vi "FetchSettings.vi"(3 "error in (no error)":errorcluster, 5 "resource name 5112":refnum<k15>) -> (0 "error out (no error)":errorcluster, 1 "DataOut":string)   [LabVIEW 2011]
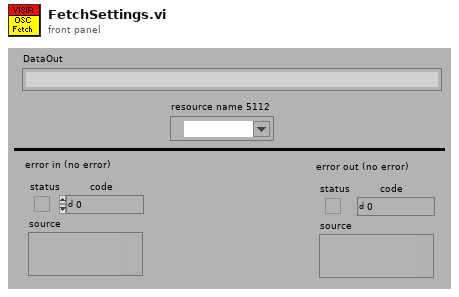
[diagram p1: front panel]
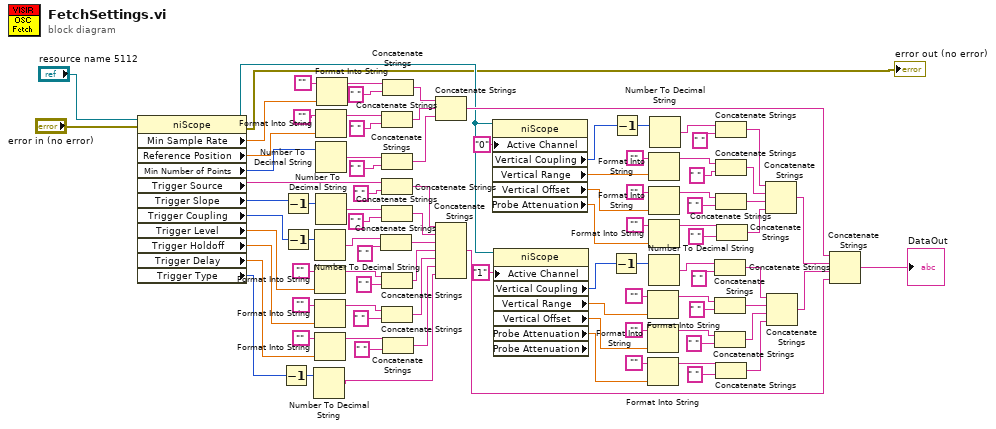
[diagram p0: block diagram]
diagram:
  n1 = property class="niScope"(reference="resource name 5112", error in="error in (no error)") -> (reference out=w9:refnum<k15>, error out=→"error out (no error)":errorcluster, "Min Sample Rate"=w89:dbl, "Reference Position"=w88:dbl, "Min Number of Points"=w86:i32, "Trigger Source"=w84:string, "Trigger Slope"=w66:i32, "Trigger Coupling"=w64:i32, "Trigger Level"=w70:dbl, "Trigger Holdoff"=w69:dbl, "Trigger Delay"=w68:dbl, "Trigger Type"=w62:i32)
  n2 = Decrement(x=w62) -> (x-1=w63:i32)
  n3 = Decrement(x=w66) -> (x-1=w67:i32)
  n4 = Decrement(x=w64) -> (x-1=w65:i32)
  n5 = Number To Decimal String(number=w63) -> (decimal integer string=w5:string)  [unwired: 1 in]
  n6 = Number To Decimal String(number=w65) -> (decimal integer string=w80:string)  [unwired: 1 in]
  n7 = Format Into String(initial string="", w70) -> (resulting string=w73:string)  [unwired: 2 in, 1 out]
  n8 = Format Into String(initial string="", w69) -> (resulting string=w71:string)  [unwired: 2 in, 1 out]
  n9 = Format Into String(initial string="", w68) -> (resulting string=w75:string)  [unwired: 2 in, 1 out]
  n10 = Format Into String(initial string="", w88) -> (resulting string=w90:string)  [unwired: 2 in, 1 out]
  n11 = Number To Decimal String(number=w86) -> (decimal integer string=w87:string)  [unwired: 1 in]
  n12 = Number To Decimal String(number=w67) -> (decimal integer string=w81:string)  [unwired: 1 in]
  n13 = Format Into String(initial string="", w89) -> (resulting string=w92:string)  [unwired: 2 in, 1 out]
  n14 = Concatenate Strings(w80, " ") -> (w45:string)
  n15 = Concatenate Strings(w90, " ") -> (w49:string)
  n16 = Concatenate Strings(w87, " ") -> (w48:string)
  n17 = Concatenate Strings(w84, " ") -> (w47:string)
  n18 = Concatenate Strings(w81, " ") -> (w46:string)
  n19 = Concatenate Strings(w73, " ") -> (w44:string)
  n20 = Concatenate Strings(w71, " ") -> (w43:string)
  n21 = Concatenate Strings(w92, " ") -> (w50:string)
  n22 = Concatenate Strings(w75, " ") -> (w42:string)
  n23 = Concatenate Strings(w50, w49, w48) -> (w41:string)
  n24 = Concatenate Strings(w47, w46, w45, w44, w43, w42, w5) -> (w18:string)
  n25 = property class="niScope"(reference=w9, "Active Channel"="0") -> ("Vertical Coupling"=w17:i32, "Vertical Range"=w16:dbl, "Vertical Offset"=w15:dbl, "Probe Attenuation"=w14:dbl)  [unwired: 1 in, 2 out]
  n26 = property class="niScope" props=["Active Channel", "Vertical Coupling", "Vertical Range", "Vertical Offset", "Probe Attenuation", "Probe Attenuation"](reference=w9, "Active Channel"="1") -> ("Vertical Coupling"=w13:i32, "Vertical Range"=w12:dbl, "Vertical Offset"=w11:dbl, "Probe Attenuation"=w10:dbl)  [unwired: 1 in, 3 out]
  n27 = Decrement(x=w13) -> (x-1=w29:i32)
  n28 = Decrement(x=w17) -> (x-1=w51:i32)
  n29 = Format Into String(initial string="", w12) -> (resulting string=w32:string)  [unwired: 2 in, 1 out]
  n30 = Format Into String(initial string="", w11) -> (resulting string=w30:string)  [unwired: 2 in, 1 out]
  n31 = Format Into String(initial string="", w10) -> (resulting string=w35:string)  [unwired: 2 in, 1 out]
  n32 = Format Into String(initial string="", w16) -> (resulting string=w54:string)  [unwired: 2 in, 1 out]
  n33 = Format Into String(initial string="", w15) -> (resulting string=w52:string)  [unwired: 2 in, 1 out]
  n34 = Format Into String(initial string="", w14) -> (resulting string=w57:string)  [unwired: 2 in, 1 out]
  n35 = Number To Decimal String(number=w29) -> (decimal integer string=w34:string)  [unwired: 1 in]
  n36 = Number To Decimal String(number=w51) -> (decimal integer string=w56:string)  [unwired: 1 in]
  n37 = Concatenate Strings(w34, " ") -> (w24:string)
  n38 = Concatenate Strings(w32, " ") -> (w23:string)
  n39 = Concatenate Strings(w30, " ") -> (w22:string)
  n40 = Concatenate Strings(w56, " ") -> (w28:string)
  n41 = Concatenate Strings(w54, " ") -> (w27:string)
  n42 = Concatenate Strings(w52, " ") -> (w26:string)
  n43 = Concatenate Strings(w35, " ") -> (w21:string)
  n44 = Concatenate Strings(w57, " ") -> (w25:string)
  n45 = Concatenate Strings(w28, w27, w26, w25) -> (w20:string)
  n46 = Concatenate Strings(w24, w23, w22, w21) -> (w19:string)
  n47 = Concatenate Strings(w41, w20, w19, w18) -> (→"DataOut":string)
